vi "AuMT8852B Single Payload Hopping.vi"(5 "Hopping (Hopping off)":enum16{"Hopping off", "Hopping on"}(ring), 7 "Set/Get (Set)":enum16{"Set", "Get"}(ring), 8 "error in (no error)":errorcluster, 10 "Script (3)":i32=3, 11 "VISA session":refnum<visa-resource-name>) -> (0 "error out":errorcluster, 2 "error code":i32, 3 "VISA session out":refnum<visa-resource-name>, 4 "Hopping out":enum16{"Hopping off", "Hopping on"}(ring))   [LabVIEW 2017]
doc: "Anritsu MT8850 Bluetooth Tester\n\nDetermines the Hop state setting for Bluetooth tests (Carrier, Sensitivity, etc.) whose scripts are set to Single Payload mode.\n\nINPUTS\n Set/Get - whether the value is being sent to or retrieved from the instrument.\n Script - the script to access.\n Hopping - value to be used in Single Payload mode.\n\nOUTPUTS\n Hopping out - value currently being used in Single Payload mode."
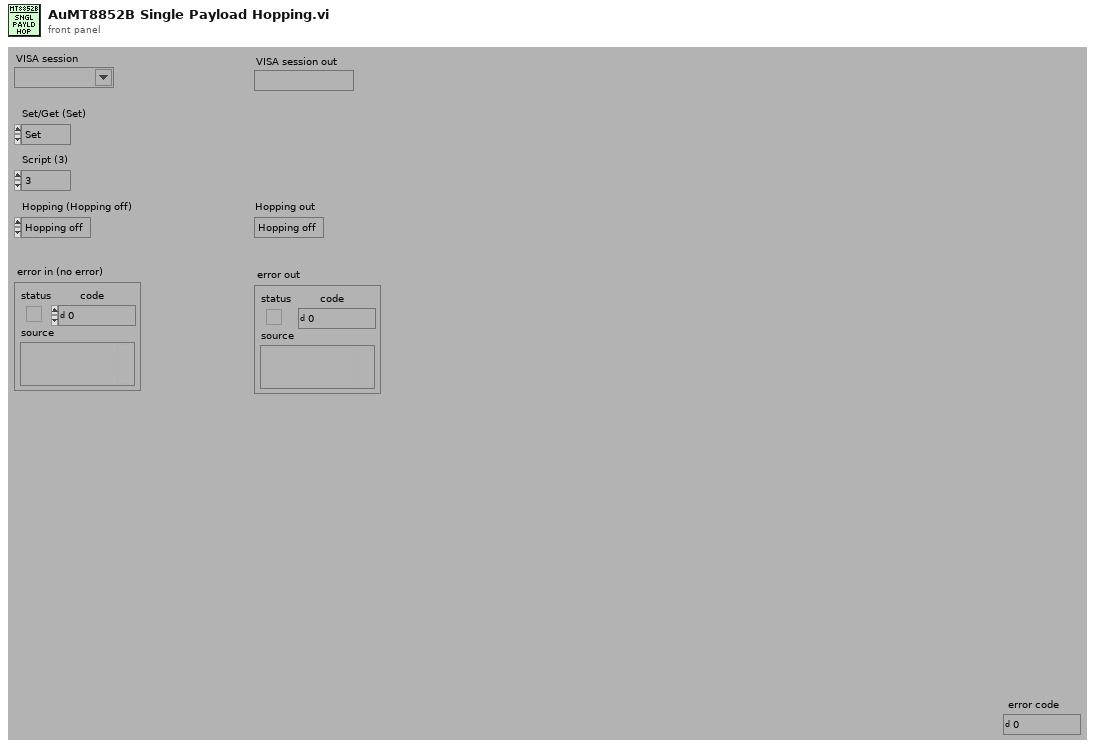
[diagram p1: front panel]
types:
  T1 = enum16{"Simulate", "Range check", "Cache", "Query instrument status"}
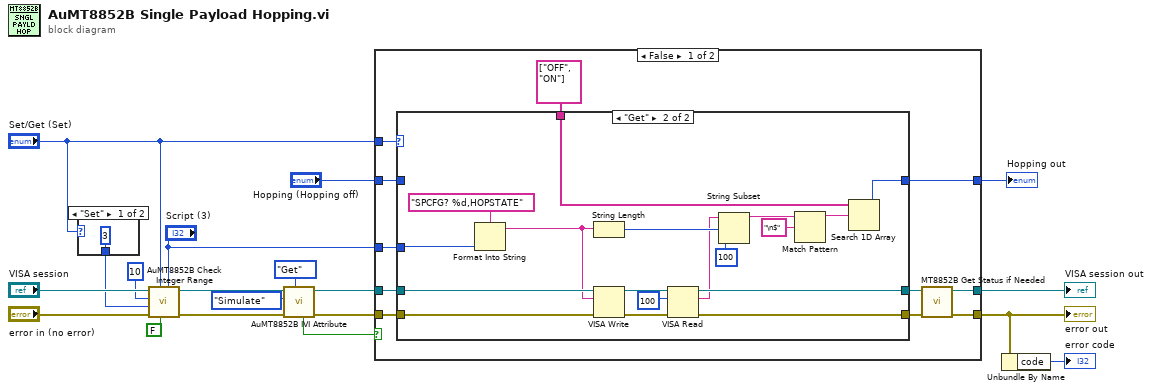
[diagram p0: block diagram]
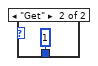
[diagram p2: hidden frame]
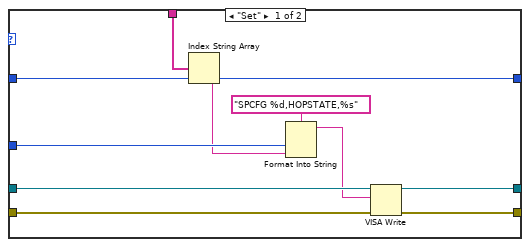
[diagram p3: hidden frame]
diagram:
  n1 = case shown="\"Set\"" "Set/Get (Set)" {
    tunnel: [3 1] -> w15
    frame "Set" {
    }
    frame "Get" {
    }
  }
  n2 = call <instrlib>:"AuMT8852B Check Integer Range.vi"("Value (0)"="Script (3)", "Check IVI flag first? (T)"=FALSE, "Set/Get (Set)"="Set/Get (Set)", "error in (no error)"="error in (no error)", "Lower limit (-1)"=w15, "Upper limit (1)"=10, "VISA session"="VISA session") -> ("error out"=w11:errorcluster, "VISA session out"=w14:refnum<visa-resource-name>)  [unwired: 3 in]
  n3 = call <instrlib>:"AuMT8852B IVI Attribute.vi"("Set/Get (Set)"=enum16{"Set", "Get"}."Get", "error in (no error)"=w11, "Flag (Simulate)"=T1."Simulate", "VISA session"=w14) -> ("error out"=w12:errorcluster, "VISA session out"=w13:refnum<visa-resource-name>, "Value out"=w8:bool)  [unwired: 5 in]
  n4 = case shown="False" w8 {
    tunnel: "Set/Get (Set)" -> [w32 _]
    tunnel: [w26 w62] -> w4
    tunnel: [w27 w63] -> w19
    tunnel: w13 -> [w31 w63]
    tunnel: w12 -> [w30 w62]
    tunnel: "Script (3)" -> [w25 _]
    tunnel: "Hopping (Hopping off)" -> [w23 w61]
    tunnel: [w22 w61] -> w1
    frame False {
      n5 = case shown="\"Get\"" w32 {
        tunnel: [w39 w54] -> w28
        tunnel: [w40 w55] -> w29
        tunnel: w31 -> [w42 w60]
        tunnel: w30 -> [w41 w59]
        tunnel: w25 -> [w36 w52]
        tunnel: string[] ["OFF", "ON"] ("Array Constant") -> [w35 w44]
        tunnel: w23 -> [w33 _]
        tunnel: [w33 w43] -> w22
        frame "Set" {
          n6 = Index String Array(1:w33, 2:w35) -> (0:w34:string)  [unwired: 1 in]
          n7 = Format Into String(format string="SPCFG %d,HOPSTATE,%s" ("Format String"), w36, w34) -> (resulting string=w37:string)  [unwired: 2 in, 1 out]
          n8 = VISA Write(VISA resource name=w42, write buffer=w37, error in (no error)=w41) -> (VISA resource name out=w40:refnum<visa-resource-name>, error out=w39:errorcluster)  [unwired: 1 out]
        }
        frame "Get" {
          n9 = Format Into String(format string="SPCFG? %d,HOPSTATE" ("Format String"), w52) -> (resulting string=w50:string)  [unwired: 2 in, 1 out]
          n10 = String Length(string=w50) -> (length=w49:i32)
          n11 = VISA Write(VISA resource name=w60, write buffer=w50, error in (no error)=w59) -> (VISA resource name out=w58:refnum<visa-resource-name>, error out=w56:errorcluster)  [unwired: 1 out]
          n12 = VISA Read(VISA resource name=w58, byte count=u32 100 ("byte count (0)"), error in (no error)=w56) -> (VISA resource name out=w55:refnum<visa-resource-name>, read buffer=w47:string, error out=w54:errorcluster)  [unwired: 1 out]
          n13 = String Subset(string=w47, offset (0)=w49, length (rest)=100 ("length (rest)")) -> (substring=w48:string)
          n14 = Match Pattern(string=w48, regular expression="\n$") -> (before substring=w45:string)  [unwired: 1 in, 3 out]
          n15 = Search 1D Array(1D array=w44, element=w45) -> (index of element=w43:i32)  [unwired: 1 in]
        }
      }
      n16 = call <instrlib>:"MT8852B Get Status if Needed.vi"("error in (no error)"=w28, "VISA session"=w29) -> ("error out"=w26:errorcluster, "VISA session out"=w27:refnum<visa-resource-name>)  [unwired: 8 in]
    }
    frame True {
    }
  }
  "error out" <- w4
  "VISA session out" <- w19
  "Hopping out" <- w1
  n17 = Unbundle By Name(w4) -> ("code"=→"error code":i32)
